vi "Finish Update.vi"(8 "instVIref":T1, 11 "target in":refnum<class "Base Target.lvclass">) -> (3 "target out":refnum<class "Base Target.lvclass">)   [LabVIEW 2020, in "NI_TargetHelper.lvlib" / "Base Target.lvclass"]
uses:
  <vilib>/TargetSupport/NI_TargetHelper/Base Target/Base Target.lvclass
  <vilib>/TargetSupport/NI_TargetHelper/Instance VIref.ctl
  <vilib>/TargetSupport/NI_TargetHelper/NI_TargetHelper.lvlib
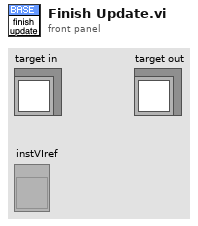
[diagram p1: front panel]
types:
  T1 = typedef "NI_TargetHelper.lvlib/Instance VIref.ctl" = refnum<vi>
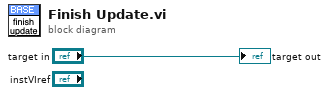
[diagram p0: block diagram]
diagram:
  "target out" <- "target in"
